vi "rad_Calculate Checksum.vi"(8 "error in":errorcluster, 9 "Ignore tmp Files":bool, 10 "List of Files to Ignore":path[](array[path]), 11 "Image Base Folder":path=path "c:/") -> (0 "error out":errorcluster, 1 "Checksums":cluster{path, "MD5 message-digest":string}[](array[cluster]), 3 "File List":path[](array[path]))   [LabVIEW 2016]
panel:
  out "Progress":i32
  out "Number of Files":i32
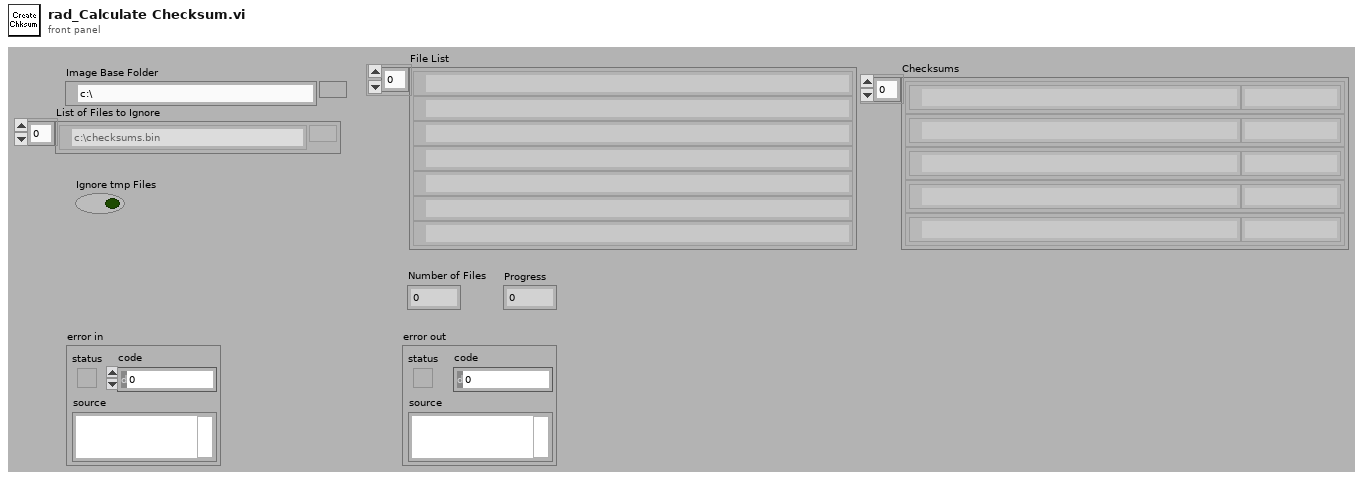
[diagram p1: front panel]
types:
  T1 = cluster{"appended path":path, "MD5 message-digest":string}
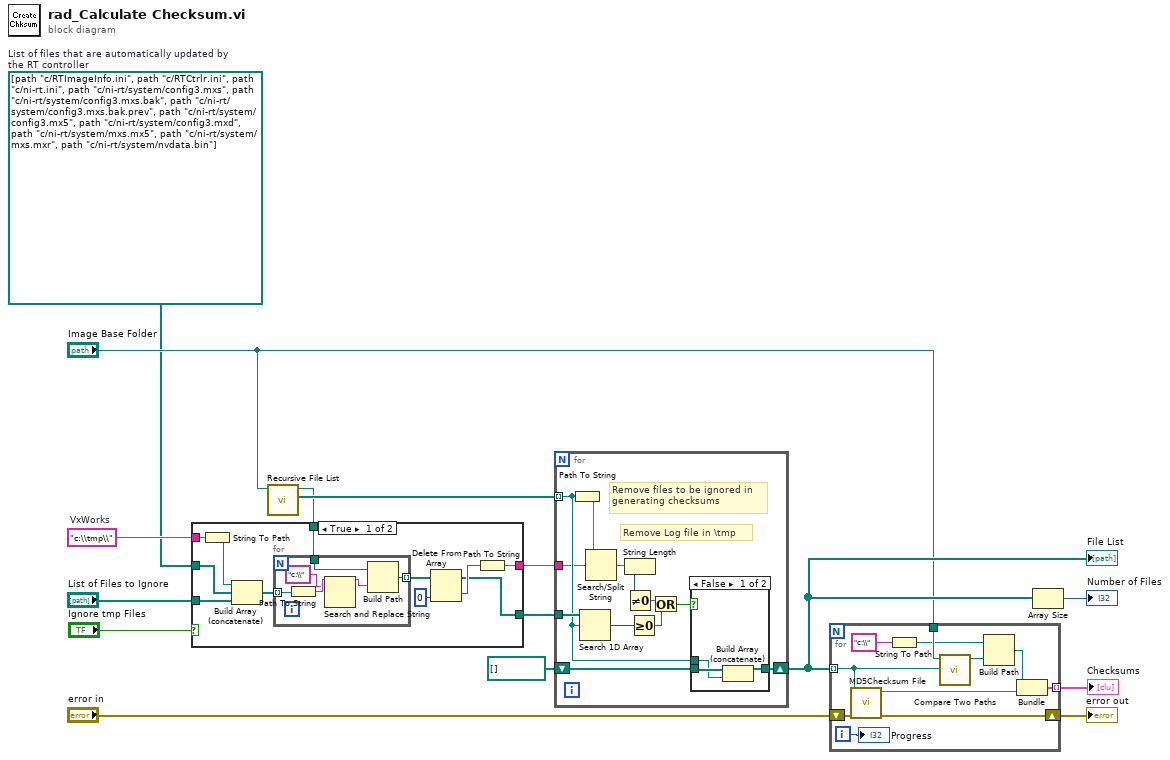
[diagram p0: block diagram]
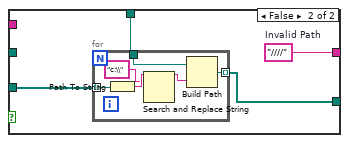
[diagram p2: hidden frame]
diagram:
  w1 = path[] [path "c:/RTImageInfo.ini", path "c:/RTCtrlr.ini", path "c:/ni-rt.ini", path "c:/ni-rt/system/config3.mxs", path "c:/ni-rt/system/config3.mxs.bak", path "c:/ni-rt/system/config3.mxs.bak.prev", path "c:/ni-rt/system/config3.mx5", path "c:/ni-rt/system/config3.mxd", path "c:/ni-rt/system/mxs.mx5", path "c:/ni-rt/system/mxs.mxr", path "c:/ni-rt/system/nvdata.bin"]  # List of files that are automatically updated by the RT controller
  w2 = "c:\\tmp\\"  # VxWorks
  n1 = call <vilib>:"Recursive File List.vi"("Folder Path"="Image Base Folder") -> ("All Files in Dir"=w9:path[], "dup Folder Path"=w8:path)  [unwired: 2 in, 7 out]
  n2 = case shown="True" "Ignore tmp Files" {
    tunnel: w8 -> [w26 w36]
    tunnel: "List of Files to Ignore" -> [w16 w35]
    tunnel: [w19 w34] -> w5
    tunnel: [w21 w33] -> w4
    tunnel: w2 -> [w20 _]
    tunnel: w1 -> [w17 _]
    frame True {
      n3 = String To Path(string=w20) -> (path=w25:path)
      n4 = Build Array (concatenate)(w25, w17, w16) -> (w24:path[])
      n5 = for {
        tunnel: w24 -> [w32] mode=indexing
        tunnel: w26 -> [w29]
        tunnel: [w27] -> w23 mode=indexing
        n6 = Path To String(path=w32) -> (string=w31:string)
        n7 = Search and Replace String(input string=w31, search string="c:\\") -> (result string=w28:string)  [unwired: 6 in, 3 out]
        n8 = Build Path(base path=w29, name or relative path=w28) -> (appended path=w27:path)
      }
      n9 = Delete From Array(array=w23, index=0) -> (deleted portion=w22:path, array with subset deleted=w19:path[])  [unwired: 1 in]
      n10 = Path To String(path=w22) -> (string=w21:string)
    }
    frame False {
      w33 = "////"  # Invalid Path
      n11 = for {
        tunnel: w35 -> [w42] mode=indexing
        tunnel: w36 -> [w39]
        tunnel: [w37] -> w34 mode=indexing
        n12 = Path To String(path=w42) -> (string=w41:string)
        n13 = Search and Replace String(input string=w41, search string="c:\\") -> (result string=w38:string)  [unwired: 6 in, 3 out]
        n14 = Build Path(base path=w39, name or relative path=w38) -> (appended path=w37:path)
      }
    }
  }
  n15 = for {
    tunnel: w9 -> [w48] mode=indexing
    shift-right: [w53] -> w12
    shift-left: path[] [] -> [w54]
    tunnel: w5 -> [w52]
    tunnel: w4 -> [w46]
    # "Remove Log file in \\tmp"
    # "Remove files to be ignored in\ngenerating checksums"
    n16 = Path To String(path=w48) -> (string=w47:string)
    n17 = Search 1D Array(1D array=w52, element=w48) -> (index of element=w51:i32)  [unwired: 1 out]
    n18 = Search/Split String(string=w47, search string/char (-)=w46) -> (match + rest of string=w45:string)  [unwired: 1 in, 2 out]
    n19 = String Length(string=w45) -> (length=w44:i32)
    n20 = Not Equal To 0?(x=w44) -> (x != 0?=w43:bool)
    n21 = Greater Or Equal To 0?(x=w51) -> (x >= 0?=w50:bool)
    n22 = Or(x=w43, y=w50) -> (x .or. y?=w49:bool)
    n23 = case shown="False" w49 {
      tunnel: [w57 w58] -> w53
      tunnel: w54 -> [w56 w58]
      tunnel: w48 -> [w55 _]
      frame False {
        n24 = Build Array (concatenate)(w56, w55) -> (w57:path[])
      }
      frame True {
      }
    }
  }
  "File List" <- w12
  n25 = for {
    tunnel: w12 -> [w64] mode=indexing
    tunnel: [w69] -> w13 mode=indexing
    shift-right: [w67] -> w7
    shift-left: "error in" -> [w68]
    tunnel: "Image Base Folder" -> [w63]
    i -> [w65]
    n26 = call <vilib>:"MD5Checksum File.vi"("error in (no error)"=w68, "Path"=w64) -> ("error out"=w67:errorcluster, "MD5 message-digest"=w66:string)  [unwired: 8 out]
    n27 = String To Path(string="c:\\") -> (path=w61:path)
    n28 = call <vilib>:"Compare Two Paths.vi"("Path 2"=w64, "Path 1"=w63) -> ("Relative Path from 1 to 2"=w60:path)  [unwired: 6 in, 3 out]
    n29 = Build Path(base path=w61, name or relative path=w60) -> (appended path=w59:path)
    n30 = Bundle("appended path"=w59, "MD5 message-digest"=w66) -> (w69:T1)  [unwired: 1 out]
    "Progress" <- w65
  }
  "error out" <- w7
  "Checksums" <- w13
  n31 = Array Size(array=w12) -> (size(s)=→"Number of Files":i32)
